vi "CoinDetectorMain.vi"() -> ()   [LabVIEW 2020]
uses:
  components/RunMeas.xctl
  <vilib>/Analysis/5stat.llb/RMS (DBL).vi
  <vilib>/Analysis/NI_AALPro.lvlib
panel:
  in  "RunMeas":dbl(xcontrol)
  in  "Tab Control":enum32{"計測", "Debug"}(tab)
  out "円":dbl
  out "現在の測定周波数 [Hz]":dbl
  out "3000 Hz":dbl
  out "4000 Hz":dbl
  out "5000 Hz":dbl
  in  "500円":dbl
  in  "100円":dbl
  in  "50円":dbl
  in  "10円":dbl
  in  "5円":dbl
  in  "1円":dbl
  out "7500 kHz":dbl
  out "6000 kHz":dbl
  out "3000 kHz":dbl
  out "Sum":dbl
  out "data 2":dynamicdata(graph) caption="コイル2次側(増幅後)"
  out "data":dynamicdata(graph) caption="コイル1次側"
  out "Freq [Hz]":dbl
  out "Freq [Hz]":dbl
  out "RMS  [mV]":dbl
  out "RMS  [mV]":dbl
  in  "stop":bool
  # "現在の周波数 [Hz]"
  # "コイル2次側の増幅後電圧（RMS）[mV]"
  # "識別結果"
  # "Fetch Count"
  # "Total Frequency"
  # "Parameters"
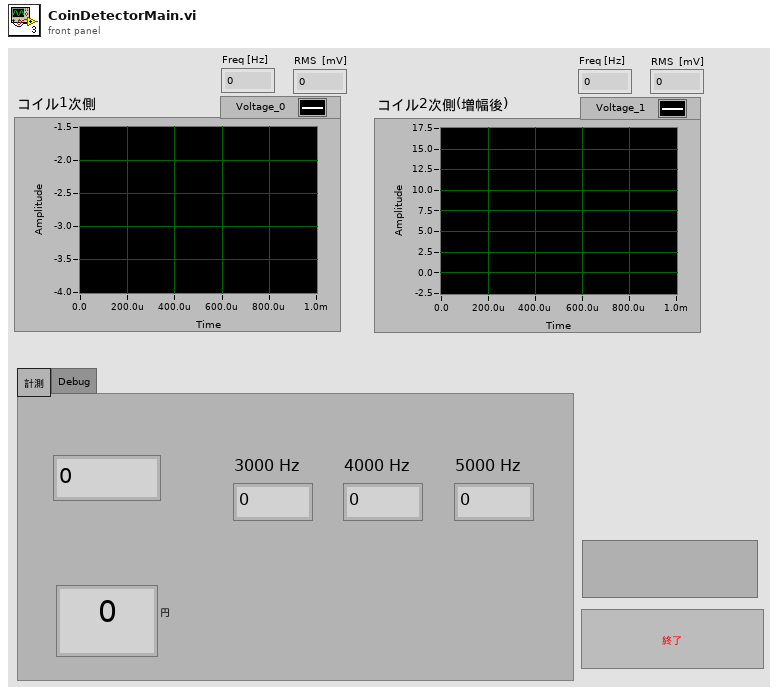
[diagram p1: front panel]
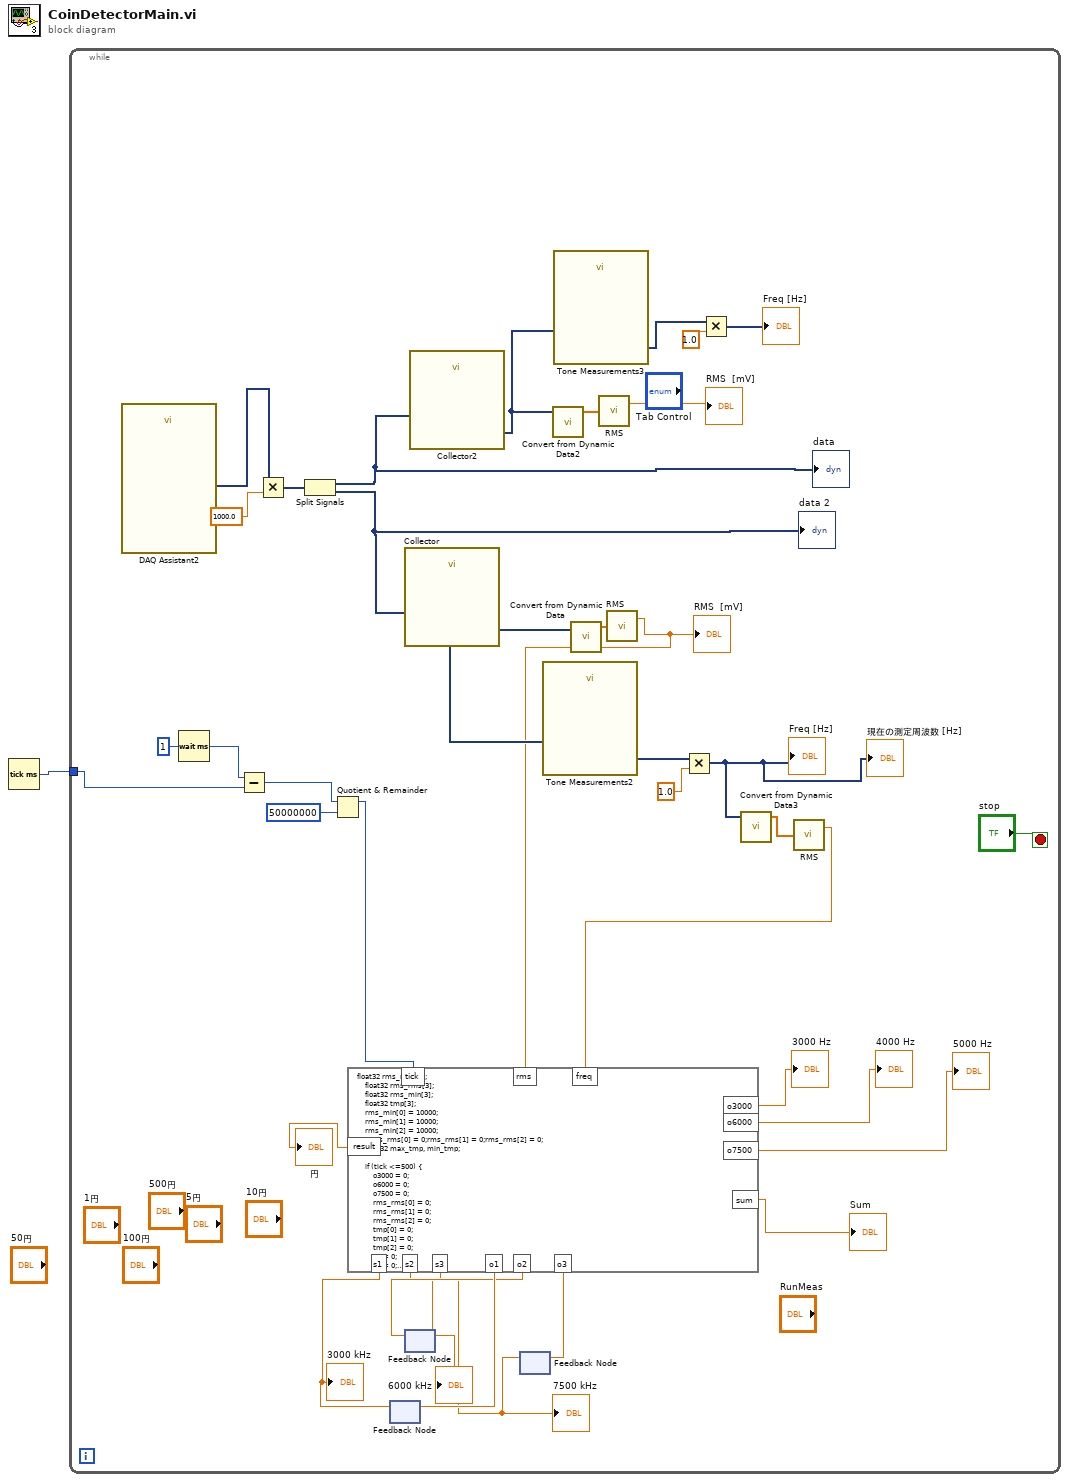
[diagram p0: block diagram]
diagram:
  n1 = Tick Count (ms)() -> (millisecond timer value=w1:u32)
  n2 = while {
    tunnel: w1 -> [w15]
    stop <- "stop" stop-if-true
    n3 = call "DAQ Assistant2"() -> ("data"=w27:dynamicdata)  [unwired: 16 in, 3 out]
    n4 = Wait (ms)(milliseconds to wait=u32 1) -> (millisecond timer value=w18:u32)
    n5 = Subtract(x=w18, y=w15) -> (x-y=w17:u32)
    n6 = Multiply(x=w27, y=1000.0) -> (x*y=w36:dynamicdata)
    n7 = Split Signals(w36) -> (w24:dynamicdata, w23:dynamicdata)  [unwired: 2 in]
    "data" <- w24
    "data 2" <- w23
    n8 = Quotient & Remainder(x=w17, y=u32 50000000) -> (x-y*floor(x/y)=w3:u32)  [unwired: 1 out]
    n9 = feedback #1() -> (w9:dbl)  [unwired: 1 in]
    "3000 kHz" <- w9
    n10 = call "Collector"("Signals"=w23) -> ("Collected Signals"=w26:dynamicdata)  [unwired: 9 in, 1 out]
    n11 = feedback #2() -> (w7:dbl)  [unwired: 1 in]
    "6000 kHz" <- w7
    n12 = call "Collector2"("Signals"=w24) -> ("Collected Signals"=w31:dynamicdata)  [unwired: 9 in, 1 out]
    n13 = feedback #3() -> (w5:dbl)  [unwired: 1 in]
    "7500 kHz" <- w5
    n14 = call "Tone Measurements2"("Signals"=w26) -> ("Frequency"=w34:dynamicdata)  [unwired: 9 in, 1 out]
    n15 = call "Convert from Dynamic Data2"("Dynamic Data Type"=w31) -> ("Array"=w33:dbl[])  [unwired: 3 in]
    n16 = call "Tone Measurements3"("Signals"=w31) -> ("Frequency"=w30:dynamicdata)  [unwired: 9 in, 1 out]
    n17 = call "Convert from Dynamic Data"("Dynamic Data Type"=w26) -> ("Array"=w35:dbl[])  [unwired: 3 in]
    n18 = call-poly <vilib>:"RMS.vi"("X"=w33) -> ("rms value"=→"RMS  [mV]":dbl)  [unwired: 1 out]
    n19 = call-poly <vilib>:"RMS.vi"("X"=w35) -> ("rms value"=w22:dbl)  [unwired: 1 out]
    "RMS  [mV]" <- w22
    n20 = Multiply(x=w34, y=1.0) -> (x*y=w4:dynamicdata)
    "Freq [Hz]" <- w4
    "現在の測定周波数 [Hz]" <- w4
    n21 = Multiply(x=w30, y=1.0) -> (x*y=→"Freq [Hz]":dynamicdata)
    n22 = call "Convert from Dynamic Data3"("Dynamic Data Type"=w4) -> ("Array"=w13:dbl[])  [unwired: 3 in]
    n23 = call-poly <vilib>:"RMS.vi"("X"=w13) -> ("rms value"=w12:dbl)  [unwired: 1 out]
    n24 = formula code="float32 rms_max[3];\n    float32 rms_rms[3];\n    float32 rms_min[3];\n    float32 tmp[3];\n    rms_min[0] = 10000;\n    rms_min[1] = 10000;\n    rms_min[2] = 10000;\n    //rms_rms[0] = 0;rms_rms[1] = 0;rms_rms[2] = 0;\n    float32 max_tmp, min_tmp;\n\n    if (tick <=500) {\n        o3000 = 0;\n        o6000 = 0;\n        o7500 = 0;\n        rms_rms[0] = 0;\n        rms_rms[1] = 0;\n        rms_rms[2] = 0;\n        tmp[0] = 0;\n        tmp[1] = 0;\n        tmp[2] = 0;\n        o1 = 0;\n        o2 = 0;\n        o3 = 0;\n    }\n\n    int32 i;\n    for (i = 0; i < 3; i++) {\n        if (i == 0) {\n            if (abs(freq - 3000) < 0.2) {\n                if (s1 >= 3 && s1 < 10) {\n                    tmp[i] = max(tmp[i], rms);\n                }\n                rms_rms[i] = tmp[i];\n                o1 = s1 + 1;\n            }\n            o3000 = rms_rms[i];\n        }\n        if (i == 1) {\n            if (abs(freq - 4000) < 0.2) {\n                if (s2 >= 3 && s2 < 10) {\n                    tmp[i] = max(tmp[i], rms);\n                }\n                rms_rms[i] = tmp[i];\n                o2 = s2 + 1;\n            }\n            o6000 = rms_rms[i];\n        }\n        if (i == 2) {\n            if (abs(freq - 5000) < 0.2) {\n                if (s3 >= 3 && s3 < 10) {\n                    tmp[i] = max(tmp[i], rms);\n                }\n                rms_rms[i] = tmp[i];\n                o3 = s3 + 1;\n            }\n            o7500 = rms_rms[i];\n        }\n    }\n    sum = o3000 + o6000 + o7500;\nif(sum>4800){\n        if(5800<=sum && sum<=6035)result=50;\n        if(6035< sum && sum<=6100)result=100;\n        if(6100< sum && sum<=6280)result=500;\n        if(6280< sum && sum<=6500)result=5;\n        if(6500< sum && sum<=6860)result=10;\n        if(6860< sum && sum<=7000)result=1;\n    }"("rms"=w22, "tick"=w3, "freq"=w12, "s1"=w9, "s2"=w7, "s3"=w5) -> ("o3000"=→"3000 Hz":dbl, "o6000"=→"4000 Hz":dbl, "o7500"=→"5000 Hz":dbl, "sum"=→"Sum":dbl, "o1"=w10:dbl, "o2"=w8:dbl, "o3"=w6:dbl, "result"=→"円":dbl)
    n25 = feedback-in #1(w10) -> ()
    n26 = feedback-in #2(w8) -> ()
    n27 = feedback-in #3(w6) -> ()
  }
